vi "Write papa Inv.vi"(8 "error in (no error)":errorcluster, 10 "Papas":i32, 11 "Productos in":refnum<class "Productos.lvclass">) -> (0 "error out":errorcluster, 3 "Productos out":refnum<class "Productos.lvclass">)   [LabVIEW 2020, in "Productos.lvlib" / "Productos.lvclass"]
uses:
  Productos.lvclass
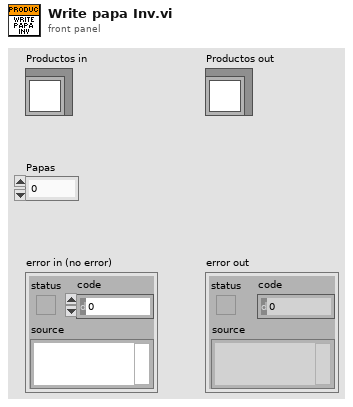
[diagram p1: front panel]
types:
  T1 = enum16{"open", "replace", "create", "open or create", "replace or create", "replace or create with confirmation"}
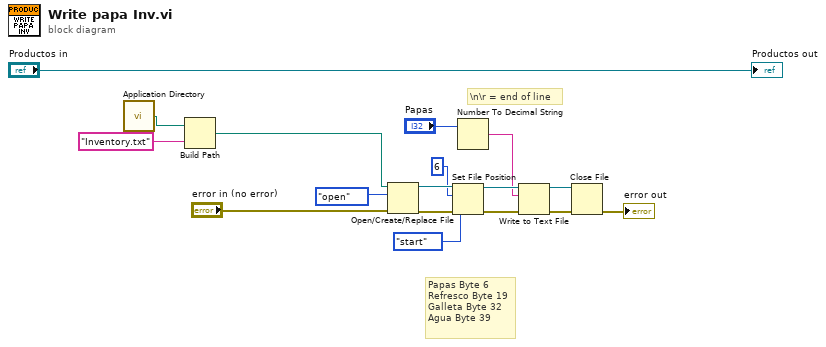
[diagram p0: block diagram]
diagram:
  # "Papas Byte 6\nRefresco Byte 19\nGalleta Byte 32\nAgua Byte 39"
  # "\\n\\r = end of line"
  n1 = call <vilib>:"Application Directory.vi"() -> ("Application Directory"=w11:path)
  n2 = Build Path(base path=w11, name or relative path="Inventory.txt" ("text")) -> (appended path=w16:path)
  n3 = Open/Create/Replace File(file path (use dialog)=w16, error in="error in (no error)", operation (0:open)=T1."open") -> (refnum out=w13:refnum<file>, error out=w15:errorcluster)  [unwired: 3 in, 1 out]
  n4 = Set File Position(offset (in bytes) (0)=i64 6, refnum=w13, from (0:start)=enum16{"start", "end", "current"}."start", error in=w15) -> (refnum out=w12:refnum<file>, error out=w10:errorcluster)
  n5 = Number To Decimal String(number="Papas") -> (decimal integer string=w1:string)  [unwired: 1 in]
  n6 = Write to Text File(file (use dialog)=w12, text=w1, error in=w10) -> (refnum out=w6:refnum<file>, error out=w7:errorcluster)  [unwired: 1 in, 1 out]
  n7 = Close File(refnum=w6, error in=w7) -> (error out=→"error out":errorcluster)  [unwired: 1 out]
  "Productos out" <- "Productos in"
